vi "niFpga wdp fft DIF 8spc.vi"(0 "real data in":fxp<+/-,8,1>[](array[numeric])=[0.0, 0.0, 0.0, 0.0, 0.0, 0.0, 0.0, 0.0], 5 "imaginary data in":fxp<+/-,8,1>[](array[numeric])=[0.0, 0.0, 0.0, 0.0, 0.0, 0.0, 0.0, 0.0], 9 "input frame start":bool, 12 "enable":bool) -> (3 "data indices":u16[](array[numeric]), 4 "real data out":fxp<+,8,1>[](array[numeric]), 6 "imaginary data out":fxp<+,8,1>[](array[numeric]), 10 "output valid":bool, 14 "ready for frame":bool, 15 "output frame start":bool)   [LabVIEW 2017]
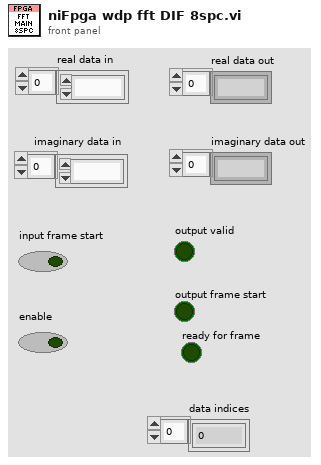
[diagram p1: front panel]
types:
  T1 = cluster{"internal input type":fxp<+/-,8,1>, "internal input type":fxp<+/-,8,1>}
  T2 = cluster{"internal input type":fxp<+/-,8,1>, "internal input type":fxp<+/-,8,1>}[]
  T3 = cluster{"x-y":fxp<+/-,20,13>, "x-y":fxp<+/-,20,13>}[]
  T4 = cluster{"data re":fxp<+/-,8,1>, "data im":fxp<+/-,8,1>}[]
  T5 = cluster{"data re":fxp<+/-,8,1>, "data im":fxp<+/-,8,1>}
  T6 = cluster{"twiddle factor type":fxp<+/-,16,2>, "twiddle factor type":fxp<+/-,16,2>}[]
  T7 = cluster{"x-y":fxp<+/-,19,12>, "x-y":fxp<+/-,19,12>}
  T8 = cluster{"x+y":fxp<+/-,19,12>, "x+y":fxp<+/-,19,12>}
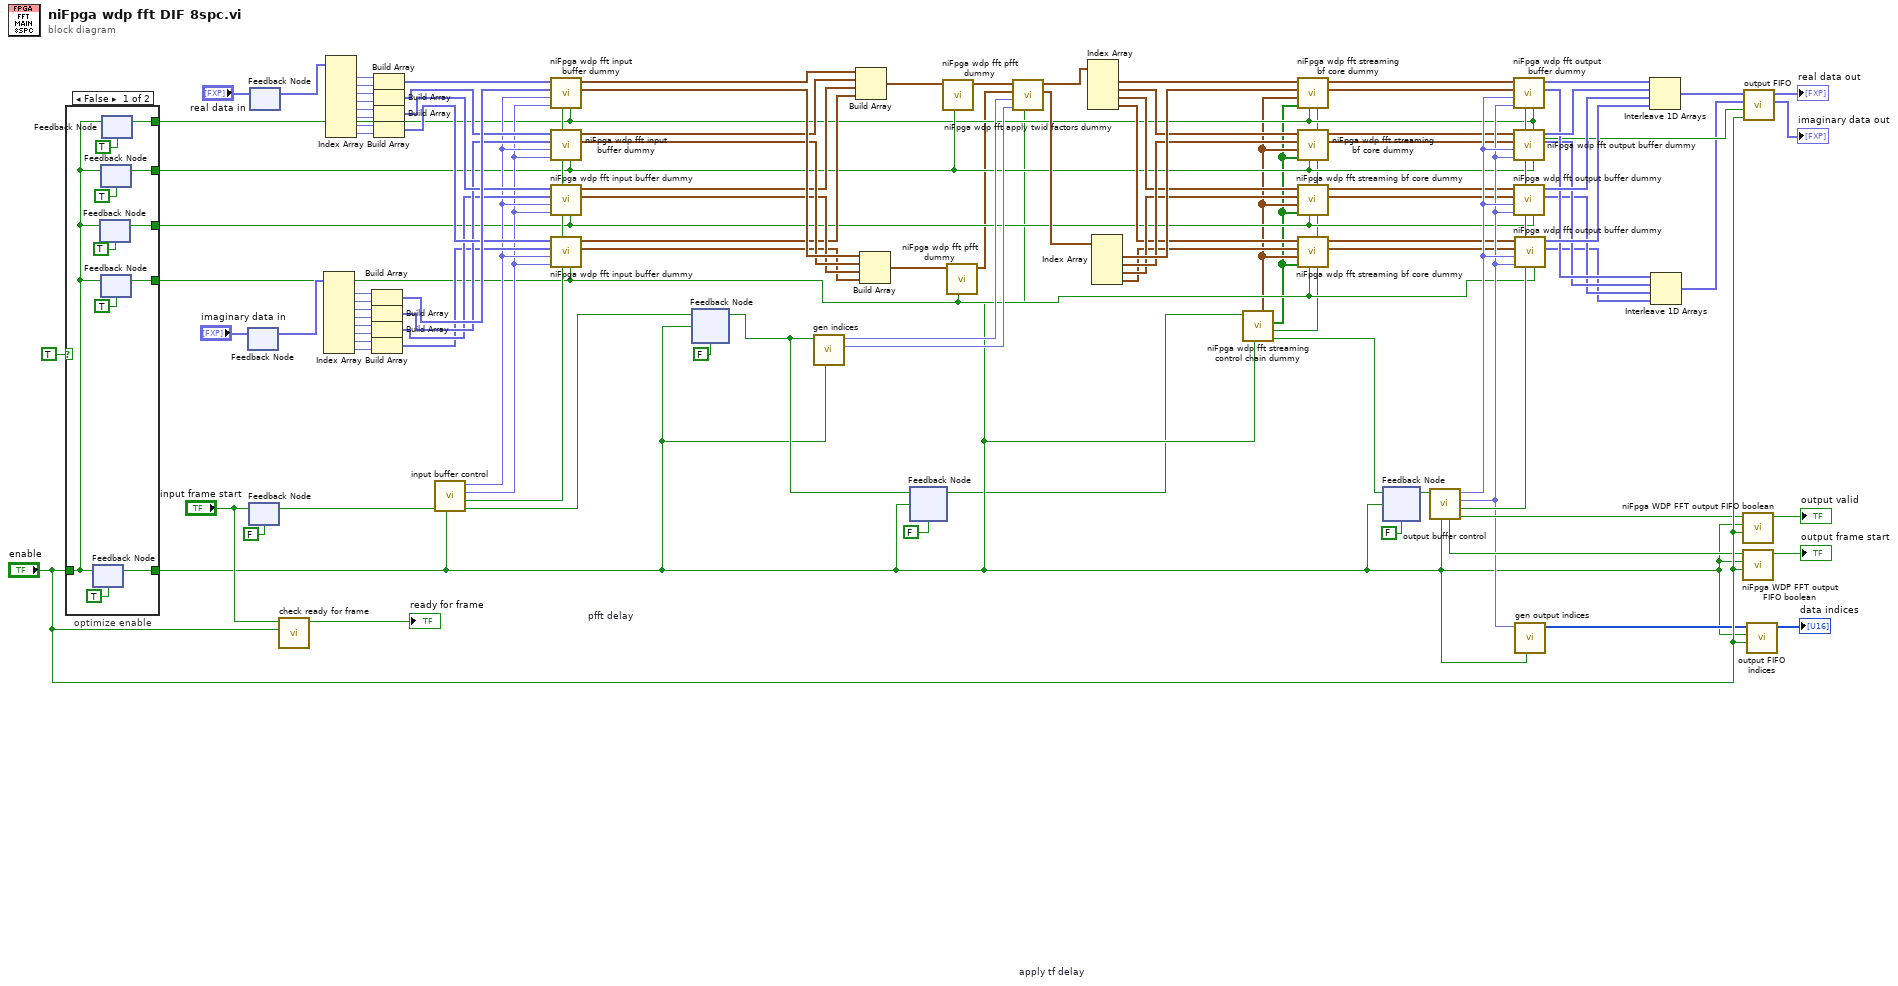
[diagram p0: block diagram]
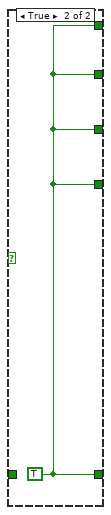
[diagram p2: hidden frame]
diagram:
  n1 = case "optimize enable" shown="False" TRUE {
    tunnel: [w117 w118] -> w32
    tunnel: [w116 w118] -> w31
    tunnel: [w115 w118] -> w30
    tunnel: [w114 w118] -> w29
    tunnel: "enable" -> [w113 _]
    tunnel: [w112 w118] -> w24
    frame False {
      n2 = feedback #1(TRUE ("enable")) -> (w112:bool)
      n3 = feedback-in #1(w113) -> ()
      n4 = feedback #2(TRUE ("enable")) -> (w116:bool)
      n5 = feedback-in #2(w113) -> ()
      n6 = feedback #3(TRUE ("enable")) -> (w117:bool)
      n7 = feedback-in #3(w113) -> ()
      n8 = feedback #4(TRUE ("enable")) -> (w115:bool)
      n9 = feedback-in #4(w113) -> ()
      n10 = feedback #5(TRUE ("enable")) -> (w114:bool)
      n11 = feedback-in #5(w113) -> ()
    }
    frame True {
      w118 = TRUE
    }
  }
  n12 = feedback #6() -> (w84:fxp<+/-,8,1>[])  [unwired: 1 in]
  n13 = feedback-in #6("imaginary data in") -> ()
  n14 = feedback #7(FALSE ("enable")) -> (w99:bool)
  n15 = feedback-in #7("input frame start") -> ()
  n16 = feedback #8() -> (w86:fxp<+/-,8,1>[])  [unwired: 1 in]
  n17 = feedback-in #8("real data in") -> ()
  n18 = call "check ready for frame"("enable"="enable", "frame start in"="input frame start") -> ("ready for frame"=→"ready for frame":bool)  [unwired: 9 in]
  n19 = Index Array(array=w84) -> (element #1=w7:fxp<+/-,8,1>, element #2=w8:fxp<+/-,8,1>, element #3=w9:fxp<+/-,8,1>, element #4=w10:fxp<+/-,8,1>, element #5=w11:fxp<+/-,8,1>, element #6=w12:fxp<+/-,8,1>, element #7=w13:fxp<+/-,8,1>, element #8=w14:fxp<+/-,8,1>)  [unwired: 8 in]
  n20 = Index Array(array=w86) -> (element #1=w22:fxp<+/-,8,1>, element #2=w21:fxp<+/-,8,1>, element #3=w20:fxp<+/-,8,1>, element #4=w19:fxp<+/-,8,1>, element #5=w18:fxp<+/-,8,1>, element #6=w17:fxp<+/-,8,1>, element #7=w16:fxp<+/-,8,1>, element #8=w15:fxp<+/-,8,1>)  [unwired: 8 in]
  n21 = Build Array(w7, w8) -> (w83:fxp<+/-,8,1>[])
  n22 = Build Array(w9, w10) -> (w73:fxp<+/-,8,1>[])
  n23 = Build Array(w11, w12) -> (w72:fxp<+/-,8,1>[])
  n24 = Build Array(w13, w14) -> (w71:fxp<+/-,8,1>[])
  n25 = Build Array(w22, w21) -> (w85:fxp<+/-,8,1>[])
  n26 = Build Array(w20, w19) -> (w82:fxp<+/-,8,1>[])
  n27 = Build Array(w18, w17) -> (w75:fxp<+/-,8,1>[])
  n28 = Build Array(w16, w15) -> (w74:fxp<+/-,8,1>[])
  n29 = call "input buffer control"("enable"=w24, "frame start in"=w99) -> ("frame start out"=w50:bool, "write memory 2?"=w64:bool, "read index"=w69:fxp<+,9,9>, "write index"=w70:fxp<+,8,8>)  [unwired: 6 in]
  n30 = call <vilib>:"niFpga wdp fft input buffer dummy.vi"("enable"=w29, "write memory 2?"=w64, "read index"=w69, "write index"=w70, "data in im"=w83, "data in re"=w85) -> ("data out 1"=w87:T1, "data out 0"=w88:T1)  [unwired: 4 in]
  n31 = call <vilib>:"niFpga wdp fft input buffer dummy.vi"("enable"=w32, "write memory 2?"=w64, "read index"=w69, "write index"=w70, "data in im"=w73, "data in re"=w82) -> ("data out 1"=w80:T1, "data out 0"=w81:T1)  [unwired: 4 in]
  n32 = call <vilib>:"niFpga wdp fft input buffer dummy.vi"("enable"=w31, "write memory 2?"=w64, "read index"=w69, "write index"=w70, "data in im"=w72, "data in re"=w75) -> ("data out 1"=w78:T1, "data out 0"=w79:T1)  [unwired: 4 in]
  n33 = call <vilib>:"niFpga wdp fft input buffer dummy.vi"("enable"=w30, "write memory 2?"=w64, "read index"=w69, "write index"=w70, "data in im"=w71, "data in re"=w74) -> ("data out 1"=w76:T1, "data out 0"=w77:T1)  [unwired: 4 in]
  n34 = feedback #9 "pfft delay"(FALSE) -> (w49:bool)
  n35 = feedback-in #9(w50, w24) -> ()
  n36 = call "gen indices"("enable"=w24, "frame start"=w49) -> ("data index 1"=w52:fxp<+,10,10>, "data index 0"=w53:fxp<+,10,10>)  [unwired: 8 in]
  n37 = Build Array(w88, w81, w79, w77) -> (w98:T2)
  n38 = Build Array(w87, w80, w78, w76) -> (w97:T2)
  n39 = feedback #10 "apply tf delay"(FALSE) -> (w23:bool)
  n40 = feedback-in #10(w49, w24) -> ()
  n41 = call <vilib>:"niFpga wdp fft pfft dummy.vi"("enable"=w32, "data in"=w98) -> ("data out"=w5:T3)  [unwired: 9 in]
  n42 = call <vilib>:"niFpga wdp fft pfft dummy.vi"("enable"=w30, "data in"=w97) -> ("data out"=w4:T3)  [unwired: 9 in]
  n43 = call <vilib>:"niFpga wdp fft apply twid factors dummy.vi"("enable"=w24, "data index 1"=w52, "data index 0"=w53, "data in 1"=w4, "data in 0"=w5) -> ("data out 1"=w105:T4, "data out 0"=w106:T4)  [unwired: 5 in]
  n44 = Index Array(array=w106) -> (element #1=w48:T5, element #2=w44:T5, element #3=w40:T5, element #4=w36:T5)  [unwired: 4 in]
  n45 = Index Array(array=w105) -> (element #1=w46:T5, element #2=w42:T5, element #3=w38:T5, element #4=w34:T5)  [unwired: 4 in]
  n46 = call <vilib>:"niFpga wdp fft streaming control chain dummy.vi"("enable"=w24, "input frame start"=w23) -> ("frame start"=w27:bool, "index=0?"=w2:bool, "switch"=w1:bool[], "twiddle factors"=w3:T6)  [unwired: 5 in, 1 out]
  n47 = call <vilib>:"niFpga wdp fft streaming bf core dummy.vi"("index=0?"=w2, "enable"=w29, "switch"=w1, "twiddle factors"=w3, "data in 1"=w46, "data in 0"=w48) -> ("data out 1"=w45:T7, "data out 0"=w47:T8)  [unwired: 4 in]
  n48 = call <vilib>:"niFpga wdp fft streaming bf core dummy.vi"("index=0?"=w2, "enable"=w32, "switch"=w1, "twiddle factors"=w3, "data in 1"=w42, "data in 0"=w44) -> ("data out 1"=w41:T7, "data out 0"=w43:T8)  [unwired: 4 in]
  n49 = call <vilib>:"niFpga wdp fft streaming bf core dummy.vi"("index=0?"=w2, "enable"=w31, "switch"=w1, "twiddle factors"=w3, "data in 1"=w38, "data in 0"=w40) -> ("data out 1"=w37:T7, "data out 0"=w39:T8)  [unwired: 4 in]
  n50 = call <vilib>:"niFpga wdp fft streaming bf core dummy.vi"("index=0?"=w2, "enable"=w30, "switch"=w1, "twiddle factors"=w3, "data in 1"=w34, "data in 0"=w36) -> ("data out 1"=w33:T7, "data out 0"=w35:T8)  [unwired: 4 in]
  n51 = feedback #11 ("delay")(FALSE) -> (w26:bool)
  n52 = feedback-in #11(w27, w24) -> ()
  n53 = call "output buffer control"("enable"=w24, "frame start"=w26) -> ("output valid?"=w60:bool, "memory switch"=w57:bool, "read index"=w56:fxp<+,4,4>, "write index"=w58:fxp<+,9,9>, "frame start?"=w59:bool)  [unwired: 5 in]
  n54 = call <vilib>:"niFpga wdp fft output buffer dummy.vi"("enable"=w29, "memory switch"=w57, "read index"=w56, "write index"=w58, "data in 1"=w45, "data in 0"=w47) -> ("data out im"=w92:fxp<+/-,32,16>[], "data out re"=w96:fxp<+/-,32,16>[])  [unwired: 4 in]
  n55 = call <vilib>:"niFpga wdp fft output buffer dummy.vi"("enable"=w32, "memory switch"=w57, "read index"=w56, "write index"=w58, "data in 1"=w41, "data in 0"=w43) -> ("data out im"=w91:fxp<+/-,32,16>[], "data out re"=w95:fxp<+/-,32,16>[])  [unwired: 4 in]
  n56 = call <vilib>:"niFpga wdp fft output buffer dummy.vi"("enable"=w31, "memory switch"=w57, "read index"=w56, "write index"=w58, "data in 1"=w37, "data in 0"=w39) -> ("data out im"=w90:fxp<+/-,32,16>[], "data out re"=w94:fxp<+/-,32,16>[])  [unwired: 4 in]
  n57 = call <vilib>:"niFpga wdp fft output buffer dummy.vi"("enable"=w30, "memory switch"=w57, "read index"=w56, "write index"=w58, "data in 1"=w33, "data in 0"=w35) -> ("data out im"=w89:fxp<+/-,32,16>[], "data out re"=w93:fxp<+/-,32,16>[])  [unwired: 4 in]
  n58 = call "gen output indices"("enable"=w24, "index"=w56) -> ("data indices"=w55:u16[])  [unwired: 9 in]
  n59 = Interleave 1D Arrays(w96, w95, w94, w93) -> (w67:fxp<+/-,32,16>[])
  n60 = Interleave 1D Arrays(w92, w91, w90, w89) -> (w25:fxp<+/-,32,16>[])
  n61 = call <vilib>:"niFpga WDP FFT output FIFO boolean.vi"("enable"="enable", "enable with delay"=w24, "boolean in"=w60) -> ("boolean out"=→"output valid":bool)  [unwired: 8 in]
  n62 = call <vilib>:"niFpga WDP FFT output FIFO boolean.vi"("enable"="enable", "enable with delay"=w24, "boolean in"=w59) -> ("boolean out"=→"output frame start":bool)  [unwired: 8 in]
  n63 = call "output FIFO"("enable"="enable", "enable with delay"=w29, "data in 1"=w25, "data in 0"=w67) -> ("data out 1"=→"imaginary data out":fxp<+,8,1>[], "data out 0"=→"real data out":fxp<+,8,1>[])  [unwired: 6 in]
  n64 = call "output FIFO indices"("enable"="enable", "enable with delay"=w24, "data in"=w55) -> ("data out"=→"data indices":u16[])  [unwired: 8 in]
